vi "Events.vi"(8 "error in (no error)":errorcluster, 11 "BasicEventLogger in":refnum<class "BasicEventLogger.lvclass">) -> (0 "error out":errorcluster, 2 "Events":T1[](array[typedef]), 3 "BasicEventLogger out":refnum<class "BasicEventLogger.lvclass">)   [LabVIEW 2020, in "Volatus.lvlib" / "BasicEventLogger.lvclass"]
uses:
  BasicEventLogger.lvclass
  Event.ctl
  Event Level.ctl
  BasicEventLogger.lvclass/BasicEventLogger.ctl
  Volatus.lvlib
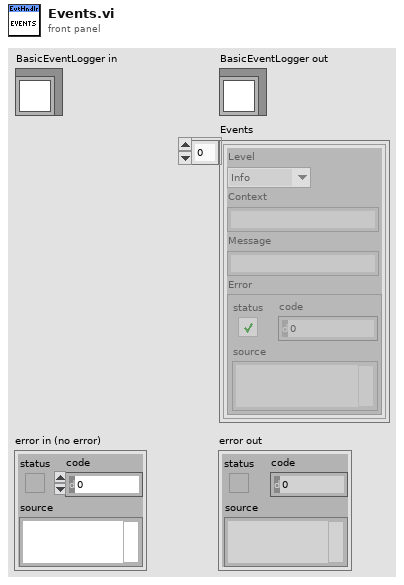
[diagram p1: front panel]
types:
  T1 = typedef "Volatus.lvlib/Event.ctl" = cluster{"Level":T2, "Context":string, "Message":string, "Error":errorcluster}
  T2 = typedef "Volatus.lvlib/Event Level.ctl" = enum16{"Debug", "Info", "Warning", "Error"}
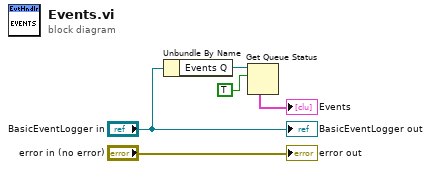
[diagram p0: block diagram]
diagram:
  n1 = Unbundle By Name("BasicEventLogger in") -> ("Events Q"=w3:refnum<queue>)
  n2 = Get Queue Status(queue=w3, return elements? (F)=TRUE) -> (elements=→"Events":T1[])  [unwired: 1 in, 7 out]
  "error out" <- "error in (no error)"
  "BasicEventLogger out" <- "BasicEventLogger in"
